vi "PYTHON Set Script Text__ogtk.vi"(4 "error in (no error)":errorcluster, 6 "script text":string, 7 "Python Session in":T1) -> (0 "error out":errorcluster, 3 "Python Session out":T1)   [LabVIEW 2017]
doc: "This function assigns the script text to the specified session. Each session can only contain one script at any one time. Assigning a new script clears any previously created script, compiled script and variable data."
uses:
  <userlib>/_OpenG.lib/labpython/labpython.llb/PYTHON Session Refnum__ogtk.ctl
  <userlib>/_OpenG.lib/labpython/lvpython.dll
panel:
  # "PYTHON Set Script Text.vi\n\nAssign the script to compile and evaluate to the session context\n\nCopyright (C) 2002 Rolf Kalbermatter rolf.kalbermatter@citeng.com\nCopyright (C) 2002 James Kring jim@jimkring.com\n\nPlease visit http://www.OpenG.org to learn about the\nOpen Source LabVIEW software movement.\n\nThis library is free software; you can redistribute it and/or\nmodify it under the terms of the GNU Lesser General Public\nLicense as published by the Free Software Foundation; either\nversion 2.1 of the License, or (at your option) any later version.\nThis library is distributed in the hope that it will be useful,\nbut WITHOUT ANY WARRANTY; without even the implied warranty of\nMERCHANTABILITY or FITNESS FOR A PARTICULAR PURPOSE. See the GNU\nLesser General Public License for more details.\nYou should have received a copy of the GNU Lesser General Public\nLicense along with this library; if not, write to the Free Software\nFoundation, Inc., 59 Temple Place, Suite 330, Boston, MA 02111-1307 USA"
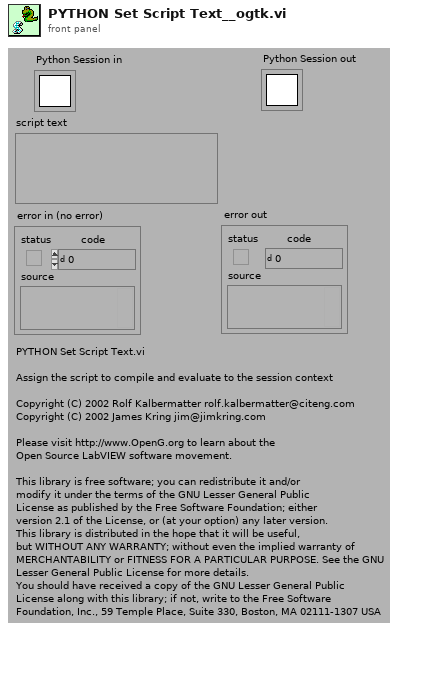
[diagram p1: front panel]
types:
  T1 = typedef "PYTHON Session Refnum__ogtk.ctl" = refnum<k1>
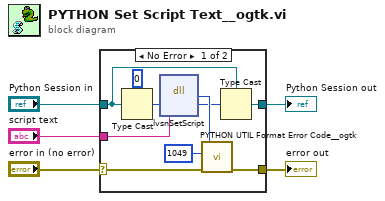
[diagram p0: block diagram]
diagram:
  n1 = case shown="No Error" "error in (no error)" {
    selector: "error in (no error)" -> [w13 w17]
    tunnel: [w7 w16] -> w1
    tunnel: [w11 w17] -> w4
    tunnel: "Python Session in" -> [w6 w16]
    tunnel: "script text" -> [w15 _]
    frame No Error {
      n2 = Type Cast(type=u32 0 ("session"), x=w6) -> (*(type *) &x=w10:u32)
      n3 = dll-call lib="C:/Program Files (x86)/National Instruments/LabVIEW 2017/user.lib/_OpenG.lib/labpython/lvpython.*" fn="lvsnSetScript"("session"=w10, "scripttext"=w15) -> (w14:i32, "session"=w8:u32)  [unwired: 4 in, 2 out]
      n4 = call <userlib>:"PYTHON UTIL Format Error Code__ogtk.vi"("error in (no error)"=w13, "code"=1049, "Bool32"=w14) -> ("error out"=w11:errorcluster)  [unwired: 4 in]
      n5 = Type Cast(type=w6, x=w8) -> (*(type *) &x=w7:T1)
    }
    frame Error {
    }
  }
  "error out" <- w4
  "Python Session out" <- w1
